vi "Configure Output.vi"(6 "Operation (0: Set Recorder Output)":i32(ring) items=["Set Recorder Output", "Set Trigger Output"], 7 "Calculate Block (1: Calculate Block 1)":i32(ring)=1 items=["Calculate Block 1"=1, "Calculate Block 2"=2, "Calculate Block 3"=3, "Calculate Block 4"=4], 8 "error in (no error)":errorcluster, 9 "Trigger Output (F: Disable)":bool, 10 "Recorder Output (F: Disable)":bool, 11 "VISA resource name":refnum<visa-resource-name>) -> (0 "error out":errorcluster, 3 "VISA resource name out":refnum<visa-resource-name>)   [LabVIEW 2018, in "Agilent U2000 Series.lvlib"]
doc: "Controls the recorder and trigger output.\n\nNote:\nThis VI supports model U2020 X-Series and U2040 X-Series only. But recorder output is not applicable for U2040 X-Series."
uses:
  Agilent U2000 Series.lvlib
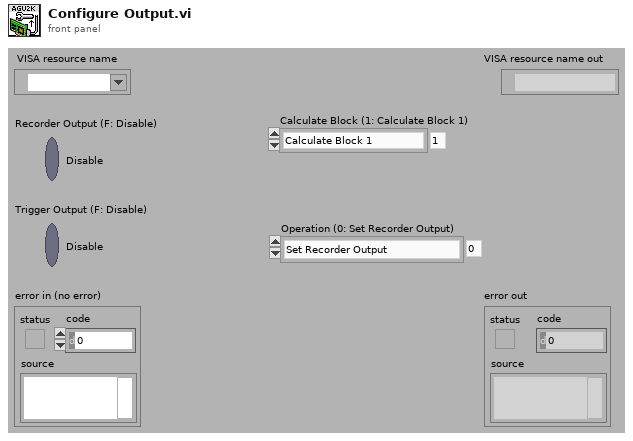
[diagram p1: front panel]
types:
  T1 = typedef "Agilent U2000 Series.lvlib/Extended User Data.ctl" = cluster{"U2000 Series Mode":u16, "Trigger Source Int/Ext":bool}
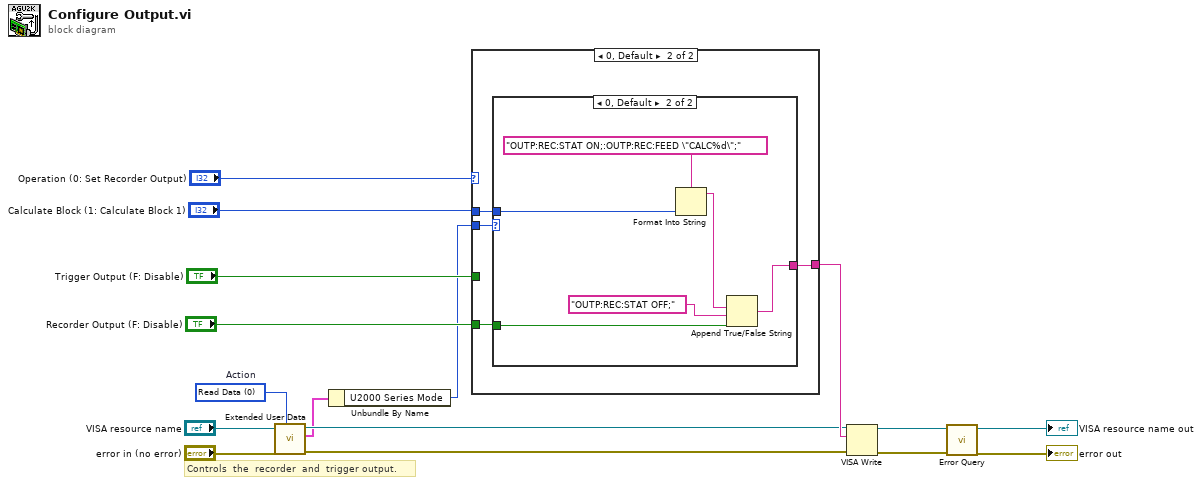
[diagram p0: block diagram]
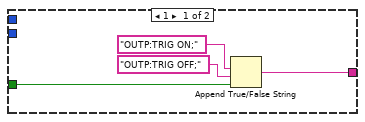
[diagram p2: hidden frame]
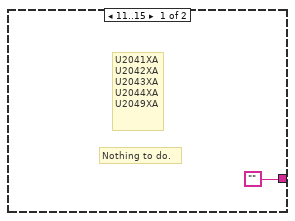
[diagram p3: hidden frame]
diagram:
  w3 = 0 items=["Read Data", "Write Data", "Clear Data", "Clear ALL Data"]  # Action
  # "Controls  the  recorder  and  trigger output."
  n1 = call "Extended User Data.vi"("Action (1: Write Data)"=w3, "error in (no error)"="error in (no error)", "VISA resource name"="VISA resource name") -> ("error out"=w4:errorcluster, "User Data Out"=w2:T1, "VISA resource name out"=w5:refnum<visa-resource-name>)  [unwired: 6 in]
  n2 = Unbundle By Name(w2) -> ("U2000 Series Mode"=w1:u16)
  n3 = case shown="0, Default" "Operation (0: Set Recorder Output)" {
    tunnel: "Recorder Output (F: Disable)" -> [_ w24]
    tunnel: "Calculate Block (1: Calculate Block 1)" -> [_ w23]
    tunnel: [w18 w22] -> w9
    tunnel: "Trigger Output (F: Disable)" -> [w17 _]
    tunnel: w1 -> [_ w21]
    frame 1 {
      n4 = Append True/False String(1:w17, 2:"OUTP:TRIG OFF;", 3:"OUTP:TRIG ON;") -> (0:w18:string)  [unwired: 1 out]
    }
    frame 0, Default {
      n5 = case shown="0, Default" w21 {
        tunnel: w24 -> [_ w30]
        tunnel: w23 -> [_ w28]
        tunnel: ["" w26] -> w22
        frame 11..15 {
          # "Nothing to do."
          # "U2041XA\nU2042XA\nU2043XA\nU2044XA\nU2049XA"
        }
        frame 0, Default {
          n6 = Format Into String(format string="OUTP:REC:STAT ON;:OUTP:REC:FEED \"CALC%d\";", w28) -> (resulting string=w27:string)  [unwired: 2 in, 1 out]
          n7 = Append True/False String(1:w30, 2:"OUTP:REC:STAT OFF;", 3:w27) -> (0:w26:string)  [unwired: 1 out]
        }
      }
    }
  }
  n8 = VISA Write(VISA resource name=w5, write buffer=w9, error in (no error)=w4) -> (VISA resource name out=w16:refnum<visa-resource-name>, error out=w15:errorcluster)  [unwired: 1 out]
  n9 = call "Error Query.vi"("error in (no error)"=w15, "VISA resource name"=w16) -> ("error out"=→"error out":errorcluster, "VISA resource name out"=→"VISA resource name out":refnum<visa-resource-name>)  [unwired: 8 out]
